vi "Double Encoder.vi"(9 "Array In":u8[](array[numeric]), 10 "Key":u32, 11 "Value":dbl) -> (1 "Array":u8[](array[numeric]))   [LabVIEW 2016]
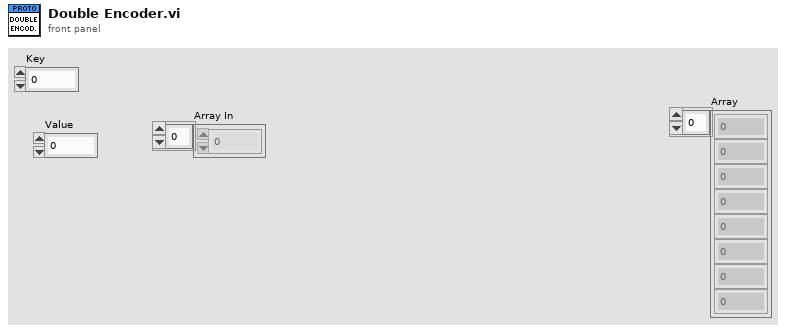
[diagram p1: front panel]
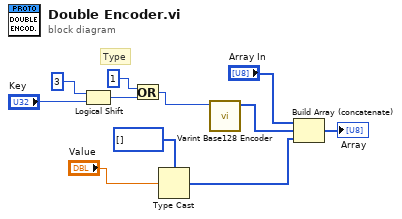
[diagram p0: block diagram]
diagram:
  # "Type"
  n1 = Logical Shift(y=i16 3, x="Key") -> (x << y=w9:u32)
  n2 = Or(x=u32 1, y=w9) -> (x .or. y?=w7:u32)
  n3 = Type Cast(type=u8[] [], x="Value") -> (*(type *) &x=w2:u8[])
  n4 = call "Varint Base128 Encoder.vi"("Numeric"=w7) -> ("Array"=w6:u8[])  [unwired: 10 in]
  n5 = Build Array (concatenate)("Array In", w6, w2) -> (→"Array":u8[])
